vi "HandleObservation.vi"(8 "error in (no error)":errorcluster, 11 "S4ACS_GUI in":refnum<class "S4GUI.lvclass">) -> (0 "error out":errorcluster, 3 "S4ACS_GUI out":refnum<class "S4GUI.lvclass">)   [LabVIEW 2018, in "S4GUI.lvclass"]
uses:
  S4GUI.lvclass
  S4GUI.lvclass/S4GUI.ctl
  Acquisition/Acquisition.lvclass
  Trigger/Trigger.lvclass
  SyncBox/Sync Box.lvclass
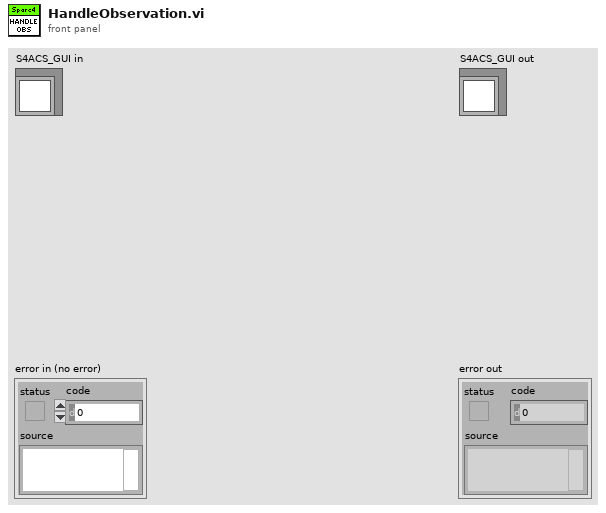
[diagram p1: front panel]
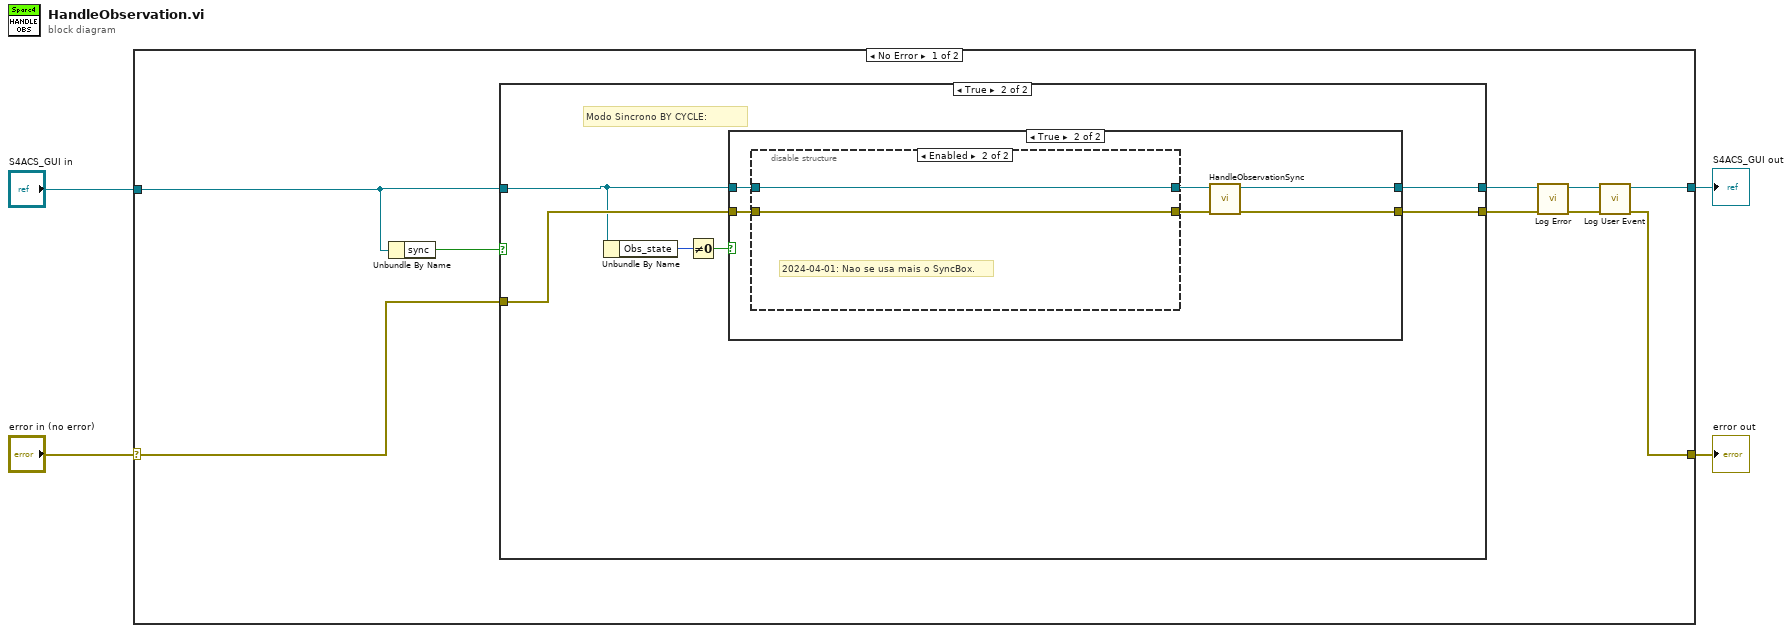
[diagram p0: block diagram]
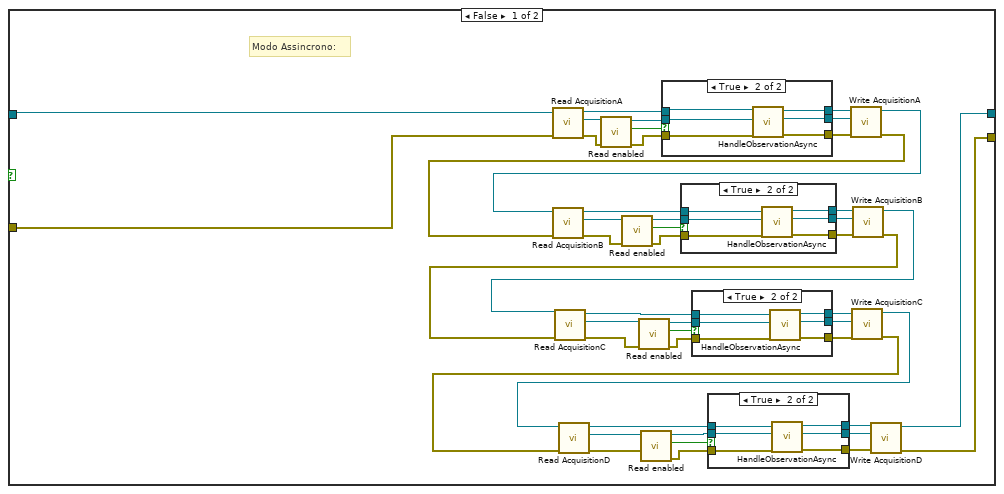
[diagram p2: hidden frame]
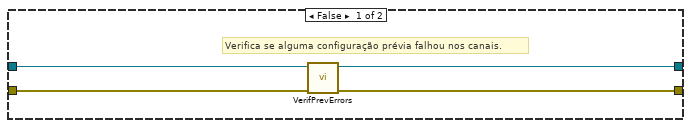
[diagram p7: hidden frame]
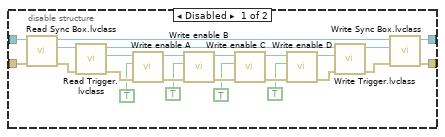
[diagram p8: hidden frame]
diagram:
  n1 = case shown="No Error" "error in (no error)" {
    selector: "error in (no error)" -> [w11 w139]
    tunnel: [w5 w139] -> w3
    tunnel: [w6 w138] -> w1
    tunnel: "S4ACS_GUI in" -> [w13 w138]
    frame No Error {
      n2 = Unbundle By Name(w13) -> ("sync"=w12:bool)
      n3 = case shown="True" w12 {
        tunnel: w13 -> [w21 w98]
        tunnel: [w55 w101] -> w10
        tunnel: w11 -> [w20 w99]
        tunnel: [w54 w100] -> w9
        frame False {
          # "Modo Assincrono:"
          n4 = call-dynamic "Read AcquisitionA.vi"("error in (no error)"=w20, "S4ACS_GUI in"=w21) -> ("error out"=w50:errorcluster, "Acquisition.lvclass"=w53:refnum<class "Acquisition.lvclass">, "S4ACS_GUI out"=w59:refnum<class "S4GUI.lvclass">)  [unwired: 7 in]
          n5 = call-dynamic "Read enabled.vi"("error in (no error)"=w50, "Server in"=w53) -> ("error out"=w49:errorcluster, "enabled"=w51:bool, "Server out"=w52:refnum<class "Acquisition.lvclass">)  [unwired: 7 in]
          n6 = case shown="True" w51 {
            tunnel: w59 -> [w88 w95]
            tunnel: w52 -> [w89 w94]
            tunnel: w49 -> [w87 w93]
            tunnel: [w88 w92] -> w58
            tunnel: [w89 w91] -> w57
            tunnel: [w87 w90] -> w56
            frame False {
            }
            frame True {
              n7 = call-dynamic "HandleObservationAsync.vi"("error in (no error)"=w93, "Acquisition.lvclass In"=w94, "S4ACS_GUI in"=w95) -> ("error out"=w90:errorcluster, "Acquisition.lvclass Out"=w91:refnum<class "Acquisition.lvclass">, "S4ACS_GUI out"=w92:refnum<class "S4GUI.lvclass">)  [unwired: 6 in]
            }
          }
          n8 = call-dynamic "Write AcquisitionA.vi"("error in (no error)"=w56, "Acquisition.lvclass"=w57, "S4ACS_GUI in"=w58) -> ("error out"=w18:errorcluster, "S4ACS_GUI out"=w19:refnum<class "S4GUI.lvclass">)  [unwired: 7 in]
          n9 = call "Read AcquisitionB.vi"("error in (no error)"=w18, "S4ACS_GUI in"=w19) -> ("error out"=w44:errorcluster, "Acquisition.lvclass"=w47:refnum<class "Acquisition.lvclass">, "S4ACS_GUI out"=w48:refnum<class "S4GUI.lvclass">)  [unwired: 7 in]
          n10 = call-dynamic "Read enabled.vi"("error in (no error)"=w44, "Server in"=w47) -> ("error out"=w43:errorcluster, "enabled"=w45:bool, "Server out"=w46:refnum<class "Acquisition.lvclass">)  [unwired: 7 in]
          n11 = case shown="True" w45 {
            tunnel: w48 -> [w79 w86]
            tunnel: w46 -> [w80 w85]
            tunnel: w43 -> [w78 w84]
            tunnel: [w79 w83] -> w40
            tunnel: [w80 w82] -> w41
            tunnel: [w78 w81] -> w42
            frame False {
            }
            frame True {
              n12 = call-dynamic "HandleObservationAsync.vi"("error in (no error)"=w84, "Acquisition.lvclass In"=w85, "S4ACS_GUI in"=w86) -> ("error out"=w81:errorcluster, "Acquisition.lvclass Out"=w82:refnum<class "Acquisition.lvclass">, "S4ACS_GUI out"=w83:refnum<class "S4GUI.lvclass">)  [unwired: 6 in]
            }
          }
          n13 = call "Write AcquisitionB.vi"("error in (no error)"=w42, "Acquisition.lvclass"=w41, "S4ACS_GUI in"=w40) -> ("error out"=w16:errorcluster, "S4ACS_GUI out"=w17:refnum<class "S4GUI.lvclass">)  [unwired: 7 in]
          n14 = call-dynamic "Read AcquisitionC.vi"("error in (no error)"=w16, "S4ACS_GUI in"=w17) -> ("error out"=w31:errorcluster, "Acquisition.lvclass"=w32:refnum<class "Acquisition.lvclass">, "S4ACS_GUI out"=w36:refnum<class "S4GUI.lvclass">)  [unwired: 7 in]
          n15 = call-dynamic "Read enabled.vi"("error in (no error)"=w31, "Server in"=w32) -> ("error out"=w37:errorcluster, "enabled"=w38:bool, "Server out"=w39:refnum<class "Acquisition.lvclass">)  [unwired: 7 in]
          n16 = case shown="True" w38 {
            tunnel: w36 -> [w70 w77]
            tunnel: w39 -> [w71 w76]
            tunnel: w37 -> [w69 w75]
            tunnel: [w70 w74] -> w35
            tunnel: [w71 w73] -> w34
            tunnel: [w69 w72] -> w33
            frame False {
            }
            frame True {
              n17 = call-dynamic "HandleObservationAsync.vi"("error in (no error)"=w75, "Acquisition.lvclass In"=w76, "S4ACS_GUI in"=w77) -> ("error out"=w72:errorcluster, "Acquisition.lvclass Out"=w73:refnum<class "Acquisition.lvclass">, "S4ACS_GUI out"=w74:refnum<class "S4GUI.lvclass">)  [unwired: 6 in]
            }
          }
          n18 = call-dynamic "Write AcquisitionC.vi"("error in (no error)"=w33, "Acquisition.lvclass"=w34, "S4ACS_GUI in"=w35) -> ("error out"=w14:errorcluster, "S4ACS_GUI out"=w15:refnum<class "S4GUI.lvclass">)  [unwired: 7 in]
          n19 = call-dynamic "Read AcquisitionD.vi"("error in (no error)"=w14, "S4ACS_GUI in"=w15) -> ("error out"=w26:errorcluster, "Acquisition.lvclass"=w25:refnum<class "Acquisition.lvclass">, "S4ACS_GUI out"=w27:refnum<class "S4GUI.lvclass">)  [unwired: 7 in]
          n20 = call-dynamic "Read enabled.vi"("error in (no error)"=w26, "Server in"=w25) -> ("error out"=w28:errorcluster, "enabled"=w29:bool, "Server out"=w30:refnum<class "Acquisition.lvclass">)  [unwired: 7 in]
          n21 = case shown="True" w29 {
            tunnel: w27 -> [w61 w68]
            tunnel: w30 -> [w62 w67]
            tunnel: w28 -> [w60 w66]
            tunnel: [w61 w65] -> w24
            tunnel: [w62 w64] -> w23
            tunnel: [w60 w63] -> w22
            frame False {
            }
            frame True {
              n22 = call-dynamic "HandleObservationAsync.vi"("error in (no error)"=w66, "Acquisition.lvclass In"=w67, "S4ACS_GUI in"=w68) -> ("error out"=w63:errorcluster, "Acquisition.lvclass Out"=w64:refnum<class "Acquisition.lvclass">, "S4ACS_GUI out"=w65:refnum<class "S4GUI.lvclass">)  [unwired: 6 in]
            }
          }
          n23 = call-dynamic "Write AcquisitionD.vi"("error in (no error)"=w22, "Acquisition.lvclass"=w23, "S4ACS_GUI in"=w24) -> ("error out"=w54:errorcluster, "S4ACS_GUI out"=w55:refnum<class "S4GUI.lvclass">)  [unwired: 7 in]
        }
        frame True {
          # "Modo Sincrono BY CYCLE:"
          n24 = Unbundle By Name(w98) -> ("Obs_state"=w97:u32)
          n25 = Not Equal To 0?(x=w97) -> (x != 0?=w96:bool)
          n26 = case shown="True" w96 {
            tunnel: [w103 w111] -> w101
            tunnel: [w102 w110] -> w100
            tunnel: w98 -> [w105 w109]
            tunnel: w99 -> [w104 w108]
            frame False {
              # "Verifica se alguma configuração prévia falhou nos canais."
              n27 = call-dynamic "VerifPrevErrors.vi"("error in (no error)"=w104, "S4GUI in"=w105) -> ("error out"=w102:errorcluster, "S4GUI out"=w103:refnum<class "S4GUI.lvclass">)  [unwired: 8 in]
            }
            frame True {
              n28 = disable-structure shown="Enabled" {
                disable-tunnel: w109 -> [w115 w137]
                disable-tunnel: w108 -> [w114 w136]
                disable-tunnel: [w113 w136] -> w107
                disable-tunnel: [w112 w137] -> w106
                frame Disabled {
                  n29 = call-dynamic "Read Sync Box.lvclass.vi"("error in (no error)"=w114, "SPARC4_AC in"=w115) -> ("error out"=w126:errorcluster, "Sync Box.lvclass"=w135:refnum<class "Sync Box.lvclass">, "SPARC4_AC out"=w127:refnum<class "S4GUI.lvclass">)  [unwired: 7 in]
                  n30 = call-dynamic "Read Trigger.lvclass.vi"("error in (no error)"=w126, "Sync Box in"=w135) -> ("error out"=w125:errorcluster, "Trigger.lvclass"=w134:refnum<class "Trigger.lvclass">, "Sync Box out"=w132:refnum<class "Sync Box.lvclass">)  [unwired: 7 in]
                  n31 = call "Write enable A.vi"("error in (no error)"=w125, "enable A"=TRUE, "Trigger in"=w134) -> ("error out"=w124:errorcluster, "Trigger out"=w133:refnum<class "Trigger.lvclass">)  [unwired: 7 in]
                  n32 = call "Write enable B.vi"("error in (no error)"=w124, "enable B"=TRUE, "Trigger in"=w133) -> ("error out"=w123:errorcluster, "Trigger out"=w131:refnum<class "Trigger.lvclass">)  [unwired: 7 in]
                  n33 = call "Write enable C.vi"("error in (no error)"=w123, "enable C"=TRUE, "Trigger in"=w131) -> ("error out"=w122:errorcluster, "Trigger out"=w130:refnum<class "Trigger.lvclass">)  [unwired: 7 in]
                  n34 = call "Write enable D.vi"("error in (no error)"=w122, "enable D"=TRUE, "Trigger in"=w130) -> ("error out"=w121:errorcluster, "Trigger out"=w129:refnum<class "Trigger.lvclass">)  [unwired: 7 in]
                  n35 = call-dynamic "Write Trigger.lvclass.vi"("error in (no error)"=w121, "Trigger.lvclass"=w129, "Sync Box in"=w132) -> ("error out"=w120:errorcluster, "Sync Box out"=w128:refnum<class "Sync Box.lvclass">)  [unwired: 7 in]
                  n36 = call-dynamic "Write Sync Box.lvclass.vi"("error in (no error)"=w120, "Sync Box.lvclass"=w128, "SPARC4_AC in"=w127) -> ("error out"=w113:errorcluster, "SPARC4_AC out"=w112:refnum<class "S4GUI.lvclass">)  [unwired: 7 in]
                }
                frame Enabled {
                  # "2024-04-01: Nao se usa mais o SyncBox."
                }
              }
              n37 = call-dynamic "HandleObservationSync.vi"("error in (no error)"=w107, "S4GUI in"=w106) -> ("error out"=w110:errorcluster, "S4GUI out"=w111:refnum<class "S4GUI.lvclass">)  [unwired: 8 in]
            }
          }
        }
      }
      n38 = call-dynamic "Log Error.vi"("error in (no error)"=w9, "S4GUI in"=w10) -> ("error out"=w7:errorcluster, "S4GUI out"=w8:refnum<class "S4GUI.lvclass">)  [unwired: 8 in]
      n39 = call-dynamic "Log User Event.vi"("error in (no error)"=w7, "S4GUI in"=w8) -> ("error out"=w5:errorcluster, "S4GUI out"=w6:refnum<class "S4GUI.lvclass">)  [unwired: 8 in]
    }
    frame Error {
    }
  }
  "error out" <- w3
  "S4ACS_GUI out" <- w1
